vi "Write settings.vi"(7 "force saving?":bool, 8 "error in (no error)":errorcluster, 11 "Autofocus in":refnum<class "Autofocus.lvclass">) -> (0 "error out":errorcluster, 1 "cancelled":bool, 2 "settings name":string, 3 "Autofocus out":refnum<class "Autofocus.lvclass">)   [LabVIEW 2012, in "Autofocus.lvclass"]
uses:
  Autofocus.lvclass
  <vilib>/Distrio/Murmex/Murmex/Murmex.lvclass
  Autofocus.lvclass/Autofocus.ctl
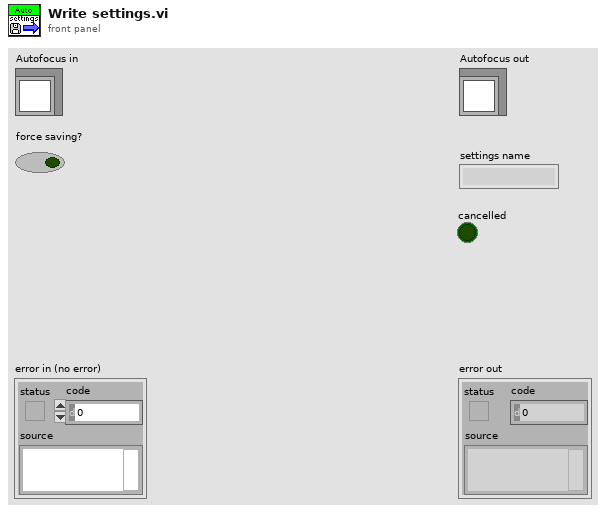
[diagram p1: front panel]
types:
  T1 = typedef "Autofocus.lvclass/settings cluster.ctl" = cluster{"Sharpness measure":T2, "ROI size":T3, "Search Algorithm":T4, "Region sampling":bool, "HC step size":dbl[unit], "current_position_focus":dbl[unit], "threshold":dbl, "brightest percentage":dbl, "number_of_checkpoints":u16, "current_stack_x":dbl[unit], "current_stack_y":dbl[unit], "curent_stack_z1":dbl[unit], "current_stack_z2":dbl[unit], "number_of_stacks":u16, "focus_start":dbl[unit], "focus_stop":dbl[unit], "frames_focus_stack":u16, "Image acquisition mode":T5, "frame rate":dbl[unit]}
  T2 = typedef "Autofocus.lvclass/Sharpness Measure.ctl" = enum16{"Vol4", "Gradient Square"}
  T3 = typedef "Autofocus.lvclass/ROI size.ctl" = u16
  T4 = typedef "Autofocus.lvclass/Search algorithm.ctl" = enum16{"Hill Climbing", "HC+GS"}
  T5 = typedef "Autofocus.lvclass/image acquisition mode.ctl" = enum16{"Focus Stack", "Single Frame"}
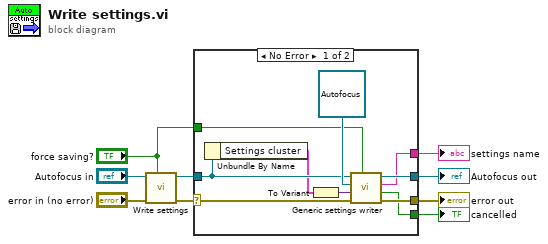
[diagram p0: block diagram]
diagram:
  n1 = call-parent "Write settings.vi"("force saving?"="force saving?", "error in (no error)"="error in (no error)", "Murmex in"="Autofocus in") -> ("error out"=w7:errorcluster, "Murmex out"=w5:refnum<class "Autofocus.lvclass">)  [unwired: 5 in, 2 out]
  n2 = case shown="No Error" w7 {
    selector: w7 -> [w19 w21]
    tunnel: [w18 w21] -> w6
    tunnel: w5 -> [w15 w20]
    tunnel: [w16 w20] -> w4
    tunnel: [w12 _] -> w3
    tunnel: [w11 _] -> w2
    tunnel: "force saving?" -> [w10 _]
    frame No Error {
      n3 = Unbundle By Name(w15) -> ("Settings cluster"=w14:T1)
      n4 = To Variant(anything=w14) -> (Variant=w13:variant)
      n5 = call <vilib>:"Generic settings writer.vi"("force saving?"=w10, "error in (no error)"=w19, "settings"=w13, "inheritance level"=refnum<class "Autofocus.lvclass"> refnum ("Autofocus.lvclass"), "Murmex in"=w15) -> ("error out"=w18:errorcluster, "cancelled"=w12:bool, "settings name"=w11:string, "Murmex out"=w16:refnum<class "Autofocus.lvclass">)  [unwired: 3 in]
    }
    frame Error {
    }
  }
  "error out" <- w6
  "Autofocus out" <- w4
  "settings name" <- w2
  "cancelled" <- w3
